vi "Auto_Gill_Configure.vi"   [LabVIEW 2010]
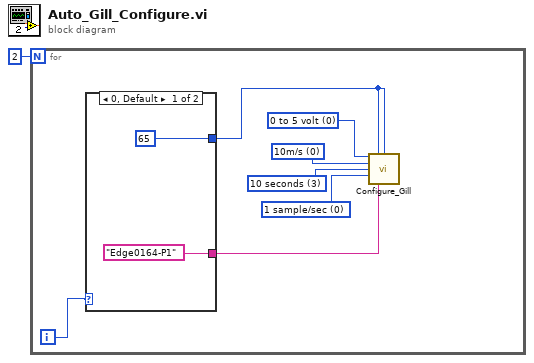
[diagram p0: block diagram]
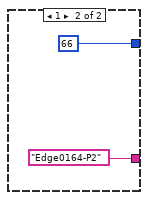
[diagram p2: hidden frame]
diagram:
  n1 = for {
    N: 2 -> [_]
    i -> [w4]
    w5 = u16 0 items=["1 sample/sec", "4 samples/sec"] ("Samples/sec")
    w6 = u16 3 items=["OFF", "3 seconds", "5 seconds", "10 seconds"] ("Averaging Time")
    w7 = u16 0 items=["10m/s", "20m/s", "30m/s", "40m/s", "50m/s", "60m/s", "70m/s"] ("Analogue O/P Scale")
    w8 = u16 0 items=["0 to 5 volt", "+/-2.5 Volt", "4-20mA"] ("Analogue O/P Config")
    n2 = case shown="0, Default" w4 {
      tunnel: ["Edge0164-P1" "Edge0164-P2"] -> w3
      tunnel: [u8 65 ("ORIGINAL Address") u8 66 ("ORIGINAL Address")] -> w2
      frame 0, Default {
      }
      frame 1 {
      }
    }
    n3 = call "Configure_Gill.vi"("Analogue O/P Config"=w8, "ORIGINAL Address"=w2, "NEW Address"=w2, "Analogue O/P Scale"=w7, "Averaging Time"=w6, "Samples/sec"=w5, "Port Name"=w3) -> ()  [unwired: 9 in]
  }
